vi "ASIOTest.vi"() -> ()   [LabVIEW 2016]
uses:
  WaveIO.dll
panel:
  in  "Device number":i32
  # "Starts the ASIO driver, extracts information and runs for 10sec\nAll output in asiotest.log"
  # "ASIO is a trademark and software of Steinberg Media Technologies GmbH"
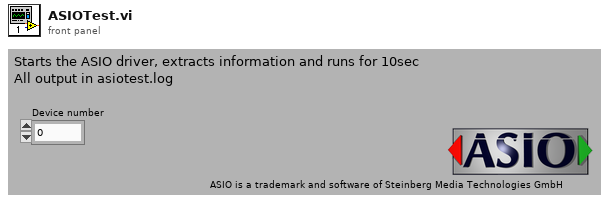
[diagram p1: front panel]
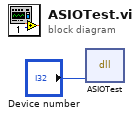
[diagram p0: block diagram]
diagram:
  n1 = dll-call lib="D:/Dokumenty/Uczelnia/LabVIEW 2/Lab2 - 09.10.2018/WaveIO/waveio.dll" fn="ASIOTest"("devnumber"="Device number") -> ()  [unwired: 5 in, 2 out]
